vi "RichToFlatcif_plugincore_StatusData.vi"(5 "OutputClusterType":T1, 11 "InputCluster":T10) -> (3 "OutputCluster":T1)   [LabVIEW 2021, in "CIF_Launcher_client.lvlib"]
uses:
  CIF_Launcher_client.lvlib
  cif_plugincore_StatusData.ctl
  cif_plugincore_StatusData_PluginState.ctl
  cif_plugincore_TimingStatistics.ctl
  cif_common_TimingStats.ctl
  cif_plugincore_FifoStatistics.ctl
  cif_plugincore_Error.ctl
  cif_plugincore_MonitorDoubles.ctl
  cif_plugincore_MonitorU64.ctl
  cif_plugincore_MonitorI64.ctl
  cif_plugincore_StatusData_Flat.ctl
  cif_plugincore_TimingStatistics_Flat.ctl
  cif_common_TimingStats_Flat.ctl
  cif_plugincore_FifoStatistics_Flat.ctl
  cif_plugincore_Error_Flat.ctl
  cif_plugincore_MonitorDoubles_Flat.ctl
  cif_plugincore_MonitorU64_Flat.ctl
  cif_plugincore_MonitorI64_Flat.ctl
  RichToFlatcif_common_TimingStats.vi
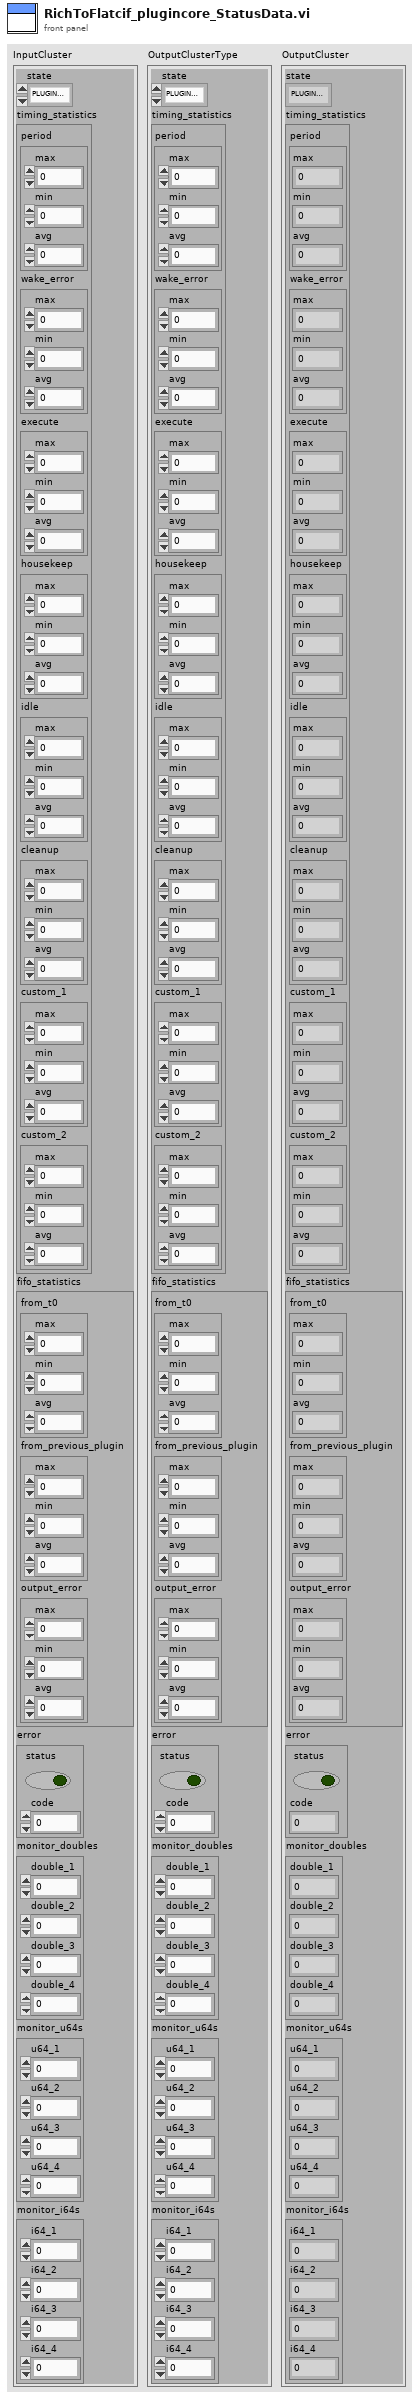
[diagram p1: front panel]
types:
  T1 = typedef "CIF_Launcher_client.lvlib/cif_plugincore_StatusData_Flat.ctl" = cluster{"state":T2, "timing_statistics":T3, "fifo_statistics":T5, "error":T6, "monitor_doubles":T7, "monitor_u64s":T8, "monitor_i64s":T9}
  T2 = typedef "CIF_Launcher_client.lvlib/cif_plugincore_StatusData_PluginState.ctl" = enum32{"PLUGINSTATE_UNKNOWN", "PLUGINSTATE_CREATING", "PLUGINSTATE_LISTENING", "PLUGINSTATE_RUNNING", "PLUGINSTATE_CLEANINGUP", "PLUGINSTATE_DESTROYING"}
  T3 = typedef "CIF_Launcher_client.lvlib/cif_plugincore_TimingStatistics_Flat.ctl" = cluster{"period":T4, "wake_error":T4, "execute":T4, "housekeep":T4, "idle":T4, "cleanup":T4, "custom_1":T4, "custom_2":T4}
  T4 = typedef "CIF_Launcher_client.lvlib/cif_common_TimingStats_Flat.ctl" = cluster{"max":i64, "min":i64, "avg":dbl}
  T5 = typedef "CIF_Launcher_client.lvlib/cif_plugincore_FifoStatistics_Flat.ctl" = cluster{"from_t0":T4, "from_previous_plugin":T4, "output_error":T4}
  T6 = typedef "CIF_Launcher_client.lvlib/cif_plugincore_Error_Flat.ctl" = cluster{"status":bool, "code":i32}
  T7 = typedef "CIF_Launcher_client.lvlib/cif_plugincore_MonitorDoubles_Flat.ctl" = cluster{"double_1":dbl, "double_2":dbl, "double_3":dbl, "double_4":dbl}
  T8 = typedef "CIF_Launcher_client.lvlib/cif_plugincore_MonitorU64_Flat.ctl" = cluster{"u64_1":u64, "u64_2":u64, "u64_3":u64, "u64_4":u64}
  T9 = typedef "CIF_Launcher_client.lvlib/cif_plugincore_MonitorI64_Flat.ctl" = cluster{"i64_1":i64, "i64_2":i64, "i64_3":i64, "i64_4":i64}
  T10 = typedef "CIF_Launcher_client.lvlib/cif_plugincore_StatusData.ctl" = cluster{"state":T2, "timing_statistics":T11, "fifo_statistics":T13, "error":T14, "monitor_doubles":T15, "monitor_u64s":T16, "monitor_i64s":T17}
  T11 = typedef "CIF_Launcher_client.lvlib/cif_plugincore_TimingStatistics.ctl" = cluster{"period":T12, "wake_error":T12, "execute":T12, "housekeep":T12, "idle":T12, "cleanup":T12, "custom_1":T12, "custom_2":T12}
  T12 = typedef "CIF_Launcher_client.lvlib/cif_common_TimingStats.ctl" = cluster{"max":i64, "min":i64, "avg":dbl}
  T13 = typedef "CIF_Launcher_client.lvlib/cif_plugincore_FifoStatistics.ctl" = cluster{"from_t0":T12, "from_previous_plugin":T12, "output_error":T12}
  T14 = typedef "CIF_Launcher_client.lvlib/cif_plugincore_Error.ctl" = cluster{"status":bool, "code":i32}
  T15 = typedef "CIF_Launcher_client.lvlib/cif_plugincore_MonitorDoubles.ctl" = cluster{"double_1":dbl, "double_2":dbl, "double_3":dbl, "double_4":dbl}
  T16 = typedef "CIF_Launcher_client.lvlib/cif_plugincore_MonitorU64.ctl" = cluster{"u64_1":u64, "u64_2":u64, "u64_3":u64, "u64_4":u64}
  T17 = typedef "CIF_Launcher_client.lvlib/cif_plugincore_MonitorI64.ctl" = cluster{"i64_1":i64, "i64_2":i64, "i64_3":i64, "i64_4":i64}
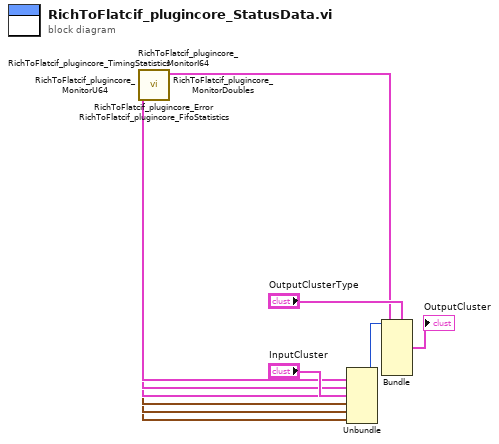
[diagram p0: block diagram]
diagram:
  n1 = Unbundle "Unbundle"("InputCluster") -> ("state"=w13:T2, "timing_statistics"=w12:T11, "fifo_statistics"=w10:T13, "error"=w8:T14, "monitor_doubles"=w6:T15, "monitor_u64s"=w4:T16, "monitor_i64s"=w2:T17)
  n2 = call "RichToFlatcif_plugincore_MonitorI64.vi"("InputCluster"=w2) -> ("OutputCluster"=w1:T9)  [unwired: 10 in]
  n3 = call "RichToFlatcif_plugincore_MonitorU64.vi"("InputCluster"=w4) -> ("OutputCluster"=w3:T8)  [unwired: 10 in]
  n4 = call "RichToFlatcif_plugincore_MonitorDoubles.vi"("InputCluster"=w6) -> ("OutputCluster"=w5:T7)  [unwired: 10 in]
  n5 = call "RichToFlatcif_plugincore_Error.vi"("InputCluster"=w8) -> ("OutputCluster"=w7:T6)  [unwired: 10 in]
  n6 = call "RichToFlatcif_plugincore_FifoStatistics.vi"("InputCluster"=w10) -> ("OutputCluster"=w9:T5)  [unwired: 10 in]
  n7 = call "RichToFlatcif_plugincore_TimingStatistics.vi"("InputCluster"=w12) -> ("OutputCluster"=w11:T3)  [unwired: 10 in]
  n8 = Bundle "Bundle"(cluster="OutputClusterType", "state"=w13, "timing_statistics"=w11, "fifo_statistics"=w9, "error"=w7, "monitor_doubles"=w5, "monitor_u64s"=w3, "monitor_i64s"=w1) -> (→"OutputCluster":T1)
